vi "Variant to Control Metadata.vi"(8 "error in":errorcluster, 11 "value":variant) -> (0 "error out":errorcluster, 1 "control metadata":T1, 2 "found?":bool, 3 "value out":variant)   [LabVIEW 2020, in "Value.lvlib"]
uses:
  Value.lvlib
  Control Metadata.ctl
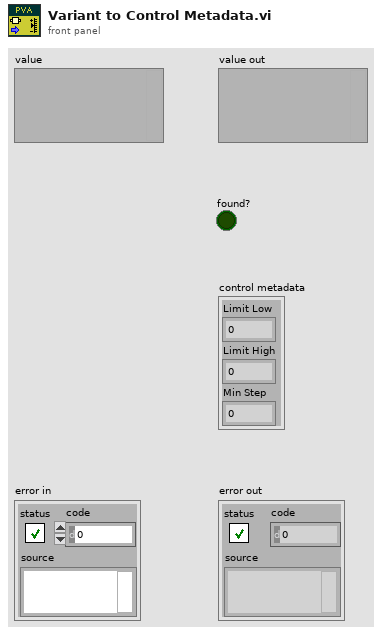
[diagram p1: front panel]
types:
  T1 = typedef "Value.lvlib/Control Metadata.ctl" = cluster{"Limit Low":dbl, "Limit High":dbl, "Min Step":dbl}
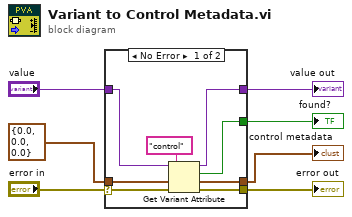
[diagram p0: block diagram]
diagram:
  n1 = case shown="No Error" "error in" {
    selector: "error in" -> [w14 w17]
    tunnel: [w11 w17] -> w7
    tunnel: "value" -> [w13 w16]
    tunnel: [w12 w16] -> w4
    tunnel: [w9 _] -> w1
    tunnel: T1 {"Limit Low"=0.0, "Limit High"=0.0, "Min Step"=0.0} ("Control Metadata") -> [w10 _]
    tunnel: [w8 _] -> w3
    frame No Error {
      n2 = Get Variant Attribute(Variant=w13, name="control", default value (empty Variant)=w10, error in=w14) -> (duplicate Variant=w12:variant, found=w8:bool, value=w9:T1, error out=w11:errorcluster)
    }
    frame Error {
    }
  }
  "error out" <- w7
  "value out" <- w4
  "found?" <- w3
  "control metadata" <- w1
